vi "SVI_extract_message_and_checksum.vi"(0 "String in":string) -> (1 "Message":string, 2 "Checksum":string)   [LabVIEW 2014]
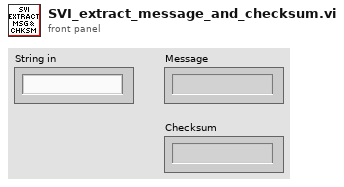
[diagram p1: front panel]
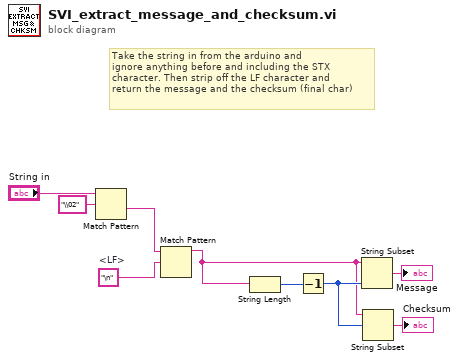
[diagram p0: block diagram]
diagram:
  w4 = "\n"  # <LF>
  # "Take the string in from the arduino and\nignore anything before and including the STX\ncharacter. Then strip off the LF character and\nreturn the message and the checksum (final char)"
  n1 = Match Pattern(string="String in", regular expression="\\02") -> (after substring=w3:string)  [unwired: 1 in, 3 out]
  n2 = Match Pattern(string=w3, regular expression=w4) -> (before substring=w7:string)  [unwired: 1 in, 3 out]
  n3 = String Length(string=w7) -> (length=w5:i32)
  n4 = Decrement(x=w5) -> (x-1=w8:i32)
  n5 = String Subset(string=w7, length (rest)=w8) -> (substring=→"Message":string)  [unwired: 1 in]
  n6 = String Subset(string=w7, offset (0)=w8) -> (substring=→"Checksum":string)  [unwired: 1 in]
